vi "Pickering 4 wire PPMS Puck 3Voltage amps.vi"(0 "26":string[](array[combo])=["NC"], 1 "27":string[](array[combo])=["NC"], 2 "28":string[](array[combo])=["NC", "NC"], 3 "1":string[](array[combo])=["NC"], 8 "5":string[](array[combo])=["NC"], 9 "4":string[](array[combo])=["NC"], 10 "3":string[](array[combo])=["NC"], 11 "2":string[](array[combo])=["NC"]) -> ()   [LabVIEW 2011]
uses:
  Lockin/source/subVI/Lock-in Globles.vi
panel:
  in  "6":string[](array[combo])=["NC"]
  in  "25":string[](array[combo])=["NC"]
  in  "24":string[](array[combo])=["NC"]
  in  "Initialize":bool
  in  "Pickering status":path=path "C:/LabView/PPMS basic VIs/Switch Status.txt"
  in  "Disconnect all?":bool
  in  "IVI Option String":string="Simulate=0,RangeCheck=1,QueryInstrStatus=0,Cache=1,DriverSetup=Model:40-726-511-M;"
  in  "VISA Resource Name":string="PXI9::13::INSTR"
  in  "X Channel Ground":string="x12"
  in  "Discharge Y Channels?":bool=TRUE
  in  "Discharge X channels?":bool=TRUE
  in  "Y Channel Ground":string="y1"
  # "4 wire              measurements\nFeature:\n1, Multiple connections\n2, Make before break\n3, First run resets device\n\nNotes:\nLock-in 1: I+/I- -->AO0/AI0, board 0\n\nLock-in 3: V+/V-  --> AI0, board 1.  \n  V+/V- conencted to y3 and y4. OSC output should set the same as Lock-in 1\n\nLock-in 2: I2+/I2- -->AO1/AI1, board 0\n\nLock-in 4: V2+/V2- -> y7/y8"
  # "2"
  # "6"
  # "25"
  # "24"
  # "5"
  # "4"
  # "3"
  # "26"
  # "27"
  # "28"
  # "1"
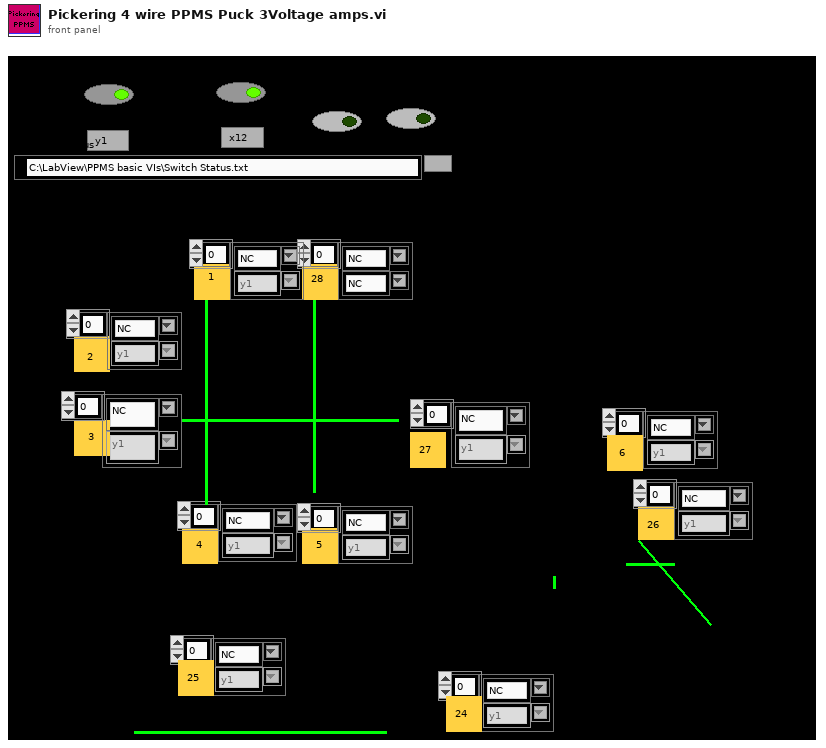
[diagram p1: front panel]
types:
  T1 = cluster{"output string":string, "output string":string}
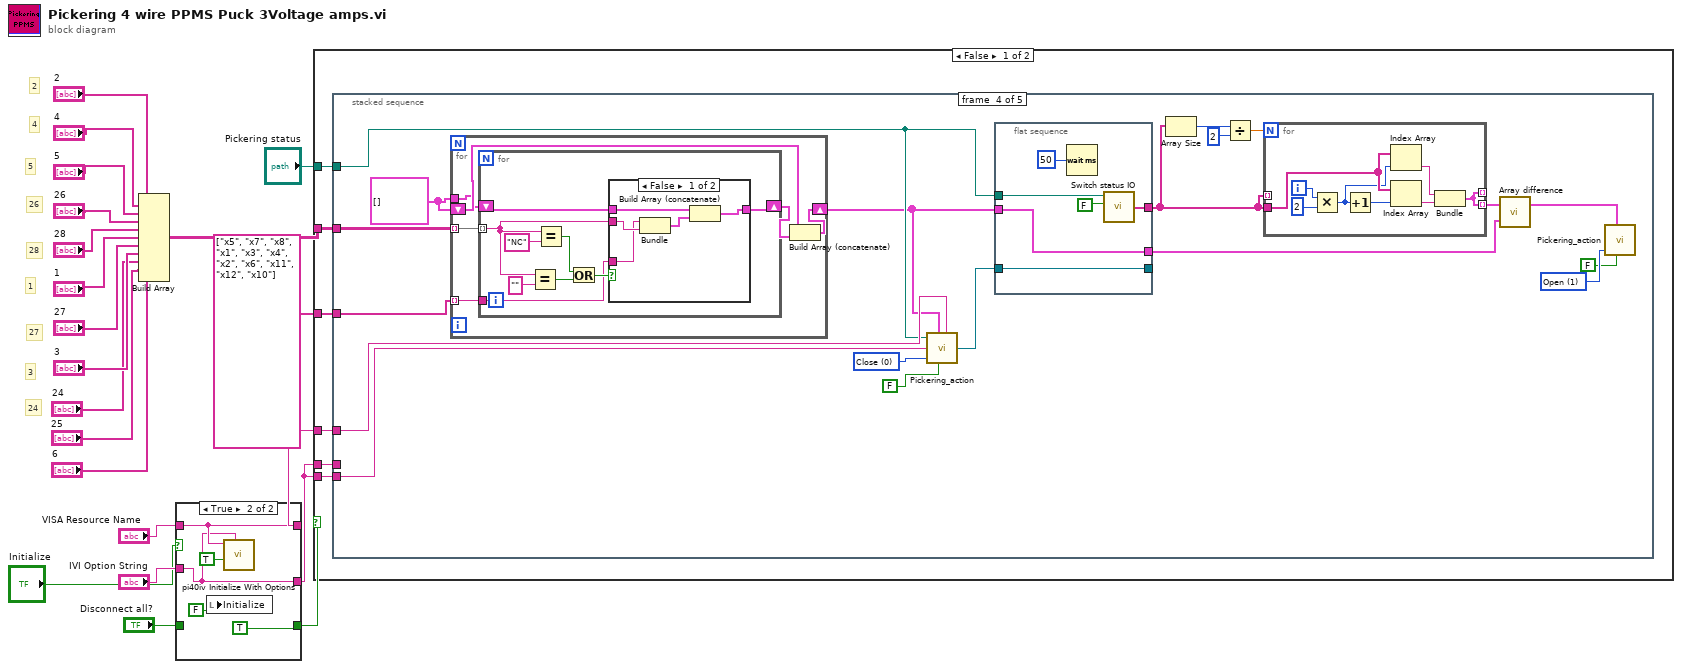
[diagram p0: block diagram]
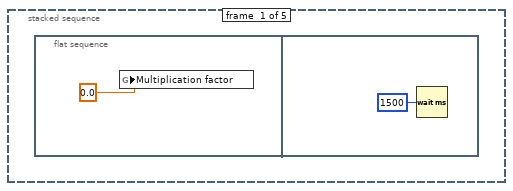
[diagram p3: hidden frame]
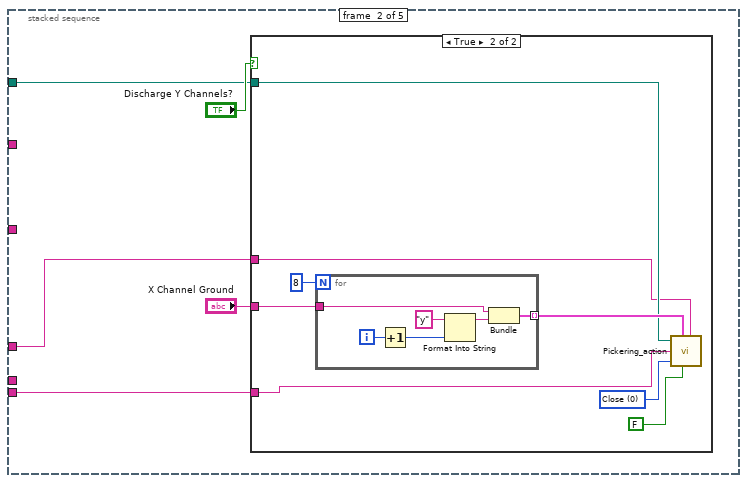
[diagram p4: hidden frame]
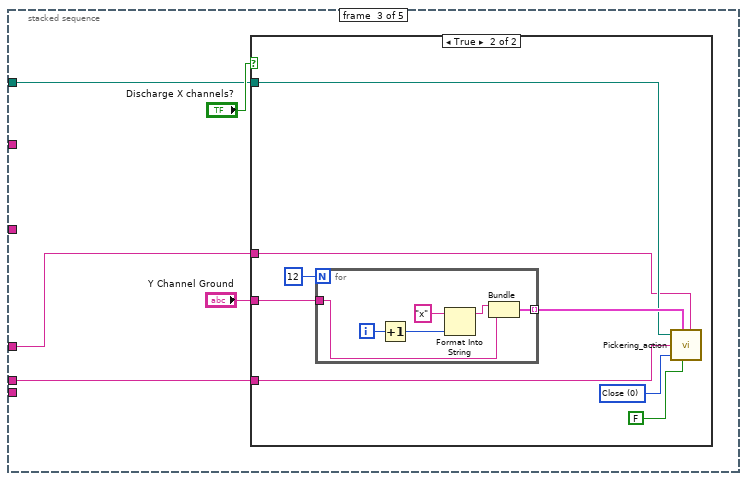
[diagram p6: hidden frame]
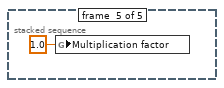
[diagram p9: hidden frame]
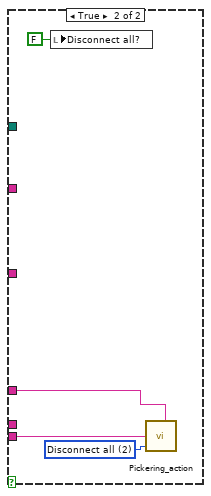
[diagram p10: hidden frame]
diagram:
  # "24"
  # "3"
  # "27"
  # "1"
  # "28"
  # "26"
  # "5"
  # "4"
  # "2"
  n1 = Build Array("2", "4", "5", "26", "28", "1", "27", "3", "24", "25", "6") -> (w19:string[][])
  n2 = case shown="True" "Initialize" {
    tunnel: "VISA Resource Name" -> [w24 w29]
    tunnel: [w24 w29] -> w17
    tunnel: "IVI Option String" -> [w23 w28]
    tunnel: [w23 w28] -> w15
    tunnel: "Disconnect all?" -> [w22 _]
    tunnel: [w22 TRUE ("reset device")] -> w12
    frame False {
    }
    frame True {
      n3 = local write "Initialize"(FALSE ("reset device")) -> ()
      n4 = call <instrlib>:"pi40iv Initialize With Options.vi"("option string"=w28, "reset device"=TRUE, "resource name"=w29) -> ()  [unwired: 7 in, 2 out]
    }
  }
  n5 = case shown="False" w12 {
    tunnel: w19 -> [w35 _]
    tunnel: string[] ["x5", "x7", "x8", "x1", "x3", "x4", "x2", "x6", "x11", "x12", "x10"] -> [w34 _]
    tunnel: w15 -> [w33 w132]
    tunnel: w17 -> [w32 w131]
    tunnel: "Pickering status" -> [w31 _]
    tunnel: w15 -> [w30 _]
    frame False {
      n6 = stacked-sequence {
        tunnel: w35 -> [_ _ _ w94 _]
        tunnel: w34 -> [_ _ _ w93 _]
        tunnel: w33 -> [_ w40 _ w92 _]
        tunnel: w32 -> [_ w38 w58 w91 _]
        tunnel: w31 -> [_ w39 w59 w90 _]
        tunnel: w30 -> [_ _ w57 _ _]
        frame #0 {
          n7 = flat-sequence {
            frame #0 {
              n8 = global write "Lock-in Globles.vi" "Multiplication factor"(0.0 ("Multiplication factor")) -> ()
            }
            frame #1 {
              n9 = Wait (ms)(milliseconds to wait=u32 1500) -> ()  [unwired: 1 out]
            }
          }
        }
        frame #1 {
          n10 = case shown="True" "Discharge Y Channels?" {
            tunnel: "X Channel Ground" -> [_ w50]
            tunnel: w40 -> [_ w46]
            tunnel: w38 -> [_ w43]
            tunnel: w39 -> [_ w45]
            frame False {
            }
            frame True {
              w47 = u16 0 items=["Close", "Open", "Disconnect all"] ("Action")
              n11 = for {
                N: 8 -> [_]
                tunnel: w50 -> [w52]
                tunnel: [w51] -> w48 mode=indexing
                i -> [w55]
                n12 = Increment(x=w55) -> (x+1=w54:i32)
                n13 = Format Into String(initial string="y", w54) -> (resulting string=w53:string)  [unwired: 2 in, 1 out]
                n14 = Bundle("X Channel Ground"=w52, w53) -> (w51:cluster{"X Channel Ground":string, string})  [unwired: 1 in]
              }
              n15 = call "Pickering_action.vi"("Pickering status"=w45, "Array"=w48, "option string"=w46, "Action"=w47, "Initialize"=FALSE, "resource name"=w43) -> ()  [unwired: 3 in, 1 out]
            }
          }
        }
        frame #2 {
          n16 = case shown="True" "Discharge X channels?" {
            tunnel: "Y Channel Ground" -> [_ w69]
            tunnel: w59 -> [_ w66]
            tunnel: w58 -> [_ w65]
            tunnel: w57 -> [_ w64]
            frame False {
            }
            frame True {
              w62 = u16 0 items=["Close", "Open", "Disconnect all"] ("Action")
              n17 = for {
                N: 12 -> [_]
                tunnel: w69 -> [w70]
                tunnel: [w72] -> w67 mode=indexing
                i -> [w74]
                n18 = Increment(x=w74) -> (x+1=w73:i32)
                n19 = Format Into String(initial string="x", w73) -> (resulting string=w71:string)  [unwired: 2 in, 1 out]
                n20 = Bundle(w71, "Y Channel Ground"=w70) -> (w72:cluster{string, "Y Channel Ground":string})  [unwired: 1 in]
              }
              n21 = call "Pickering_action.vi"("Pickering status"=w66, "Array"=w67, "option string"=w64, "Action"=w62, "Initialize"=FALSE, "resource name"=w65) -> ()  [unwired: 3 in, 1 out]
            }
          }
        }
        frame #3 {
          w81 = u16 1 items=["Close", "Open", "Disconnect all"] ("Action")
          w89 = u16 0 items=["Close", "Open", "Disconnect all"] ("Action")
          w85 = cluster{"5":string, string}[] []
          n22 = for {
            tunnel: w94 -> [w113] mode=indexing
            tunnel: w93 -> [w114] mode=indexing
            shift-right: [w112] -> w86
            shift-left: w85 -> [w110]
            tunnel: w85 -> [w109]
            n23 = for {
              tunnel: w114 -> [w118]
              tunnel: w113 -> [w117] mode=indexing
              shift-right: [w115] -> w111
              shift-left: w109 -> [w116]
              n24 = Equal?(x=w117, y="") -> (x = y?=w120:bool)
              n25 = Equal?(x=w117, y="NC") -> (x = y?=w122:bool)
              n26 = Or(x=w122, y=w120) -> (x .or. y?=w121:bool)
              n27 = case shown="False" w121 {
                tunnel: w118 -> [w124 _]
                tunnel: w117 -> [w125 _]
                tunnel: [w127 w129] -> w115
                tunnel: w116 -> [w126 w129]
                frame False {
                  n28 = Bundle(w124, "26"=w125) -> (w128:cluster{string, "26":string})  [unwired: 1 in]
                  n29 = Build Array (concatenate)(w126, w128) -> (w127:cluster{"5":string, "26":string}[])
                }
                frame True {
                }
              }
            }
            n30 = Build Array (concatenate)(w110, w111) -> (w112:cluster{"5":string, string}[])
          }
          n31 = call "Pickering_action.vi"("Pickering status"=w90, "Array"=w86, "option string"=w92, "Action"=w89, "Initialize"=FALSE, "resource name"=w91) -> ("instrument handle out"=w87:refnum<k15>)  [unwired: 3 in]
          n32 = flat-sequence {
            tunnel: w87 -> [w107]
            tunnel: [w107] -> _
            tunnel: [w106] -> w80
            tunnel: w90 -> [w105]
            tunnel: w86 -> [w103]
            tunnel: [w103] -> w78
            frame #0 {
              n33 = Wait (ms)(milliseconds to wait=u32 50) -> ()  [unwired: 1 out]
              n34 = call "Switch status IO.vi"("Write: T\nRead: F"=FALSE ("Write: T\nRead: F"), "Path"=w105) -> ("String out"=w106:string[])  [unwired: 4 in]
            }
          }
          n35 = Array Size(array=w80) -> (size(s)=w84:i32)
          n36 = Divide(x=w84, y=2) -> (x/y=w82:dbl)
          n37 = for {
            N: w82 -> [_]
            tunnel: w80 -> [w102]
            tunnel: w80 -> [_] mode=indexing
            tunnel: [w95] -> _ mode=indexing
            tunnel: [w95] -> w79 mode=indexing
            i -> [w98]
            n38 = Multiply(x=w98, y=2) -> (x*y=w96:i32)
            n39 = Increment(x=w96) -> (x+1=w101:i32)
            n40 = Index Array(array=w102, index=w96) -> (element=w100:string)
            n41 = Index Array(array=w102, index=w101) -> (element=w99:string)
            n42 = Bundle("output string"=w100, "output string"=w99) -> (w95:T1)  [unwired: 1 in]
          }
          n43 = call "Array difference.vi"("Array 2"=w78, "Array 1"=w79) -> ("Array 1-(array1&2)"=w77:cluster{"String":string, "String 2":string}[])  [unwired: 1 out]
          n44 = call "Pickering_action.vi"("Array"=w77, "Action"=w81, "Initialize"=FALSE) -> ()  [unwired: 6 in, 1 out]
        }
        frame #4 {
          n45 = global write "Lock-in Globles.vi" "Multiplication factor"(1.0 ("Multiplication factor")) -> ()
        }
      }
    }
    frame True {
      w133 = u16 2 items=["Close", "Open", "Disconnect all"] ("Action")
      n46 = local write "Disconnect all?"(FALSE ("Disconnect all?")) -> ()
      n47 = call "Pickering_action.vi"("option string"=w132, "Action"=w133, "resource name"=w131) -> ()  [unwired: 6 in, 1 out]
    }
  }
